vi "DSF.Shared.Configuration.Transfer Group.Set Timing.vi"(10 "Timing":refnum<class "DSF.Shared.Timing.lvclass">, 11 "Transfer Group Configuration in":refnum<class "DSF.Shared.Configuration.Transfer Group.lvclass">) -> (3 "Transfer Group Configuration out":refnum<class "DSF.Shared.Configuration.Transfer Group.lvclass">)   [LabVIEW 2017, in "DSF.Shared.lvlib" / "DSF.Shared.Configuration.Transfer Group.lvclass"]
uses:
  DSF.Shared.Configuration.Transfer Group.lvclass
  Timing/DSF.Shared.Timing.lvclass
  DSF.Shared.Configuration.Transfer Group.lvclass/DSF.Shared.Configuration.Transfer Group.ctl
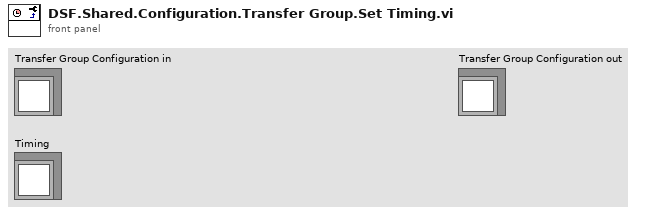
[diagram p1: front panel]
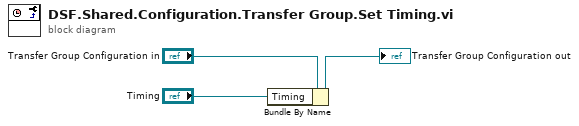
[diagram p0: block diagram]
diagram:
  n1 = Bundle By Name(cluster="Transfer Group Configuration in", "Timing"="Timing") -> (→"Transfer Group Configuration out":refnum<class "DSF.Shared.Configuration.Transfer Group.lvclass">)
